vi "Write Configure Voltage.vi"(10 "Configure Voltage":dbl, 11 "Digtal Multimeter in":refnum<class "Digital Multimeter.lvclass">) -> (3 "Digtal Multimeter out":refnum<class "Digital Multimeter.lvclass">)   [LabVIEW 2020, in "Digital Multimeter.lvclass"]
uses:
  Digital Multimeter.lvclass
  Digital Multimeter.lvclass/Digital Multimeter.ctl
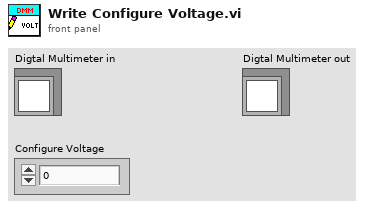
[diagram p1: front panel]
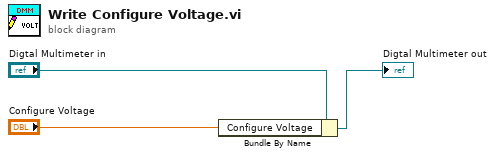
[diagram p0: block diagram]
diagram:
  n1 = Bundle By Name(cluster="Digtal Multimeter in", "Configure Voltage"="Configure Voltage") -> (→"Digtal Multimeter out":refnum<class "Digital Multimeter.lvclass">)
